vi "Initialize.vi"(8 "error in (no error)":errorcluster, 11 "WeatherSensor in":refnum<class "WeatherSensor.lvclass">) -> (0 "error out":errorcluster, 3 "WeatherSensor out":refnum<class "WeatherSensor.lvclass">)   [LabVIEW 2018, in "WeatherSensor.lvclass"]
uses:
  WeatherSensor.lvclass
  Device/Device.lvclass
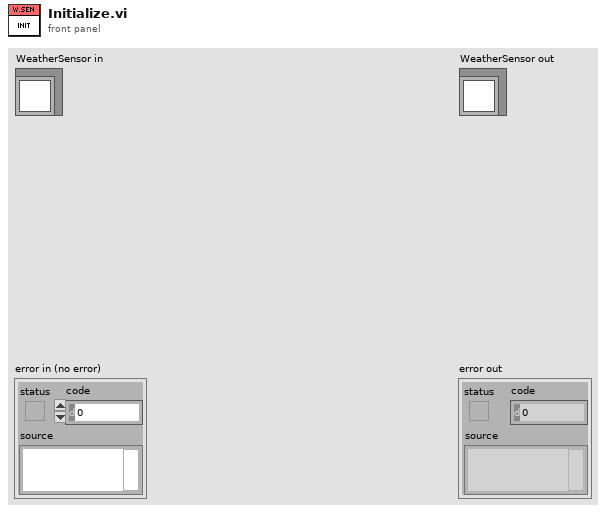
[diagram p1: front panel]
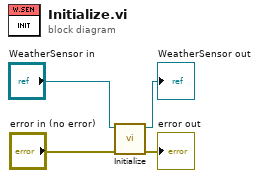
[diagram p0: block diagram]
diagram:
  n1 = call-parent "Initialize.vi"("error in (no error)"="error in (no error)", "Device in"="WeatherSensor in") -> ("error out"=→"error out":errorcluster, "Device out"=→"WeatherSensor out":refnum<class "WeatherSensor.lvclass">)  [unwired: 8 in]
